vi "Sobel.vi"() -> ()   [LabVIEW 2015]
uses:
  <vilib>/vision/NI_Vision_Development_Module.lvlib
panel:
  in  "Threshold":sgl(slide) scale=0.0..10.0
  in  "index":u8(slide) scale=-1.0..8.0
  out "Sobel":T1(plugin-control)
  out "Source":T1(plugin-control)
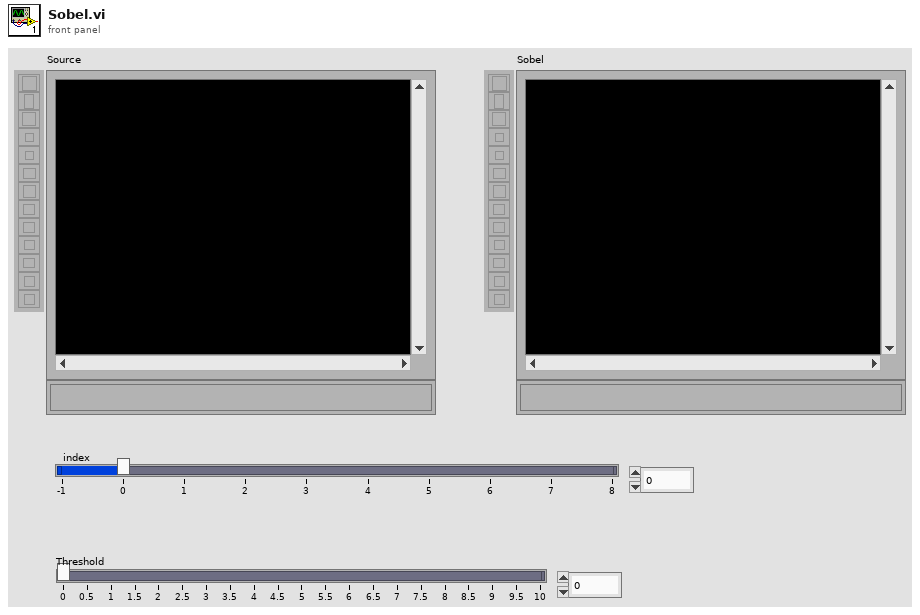
[diagram p1: front panel]
types:
  T1 = typedef "IMAQ Image.ctl" = refnum<image>
  T2 = enum32{"Differentiation", "Gradient", "Prewitt", "Roberts", "Sigma", "Sobel"}
  T3 = typedef "Image Type" = u32
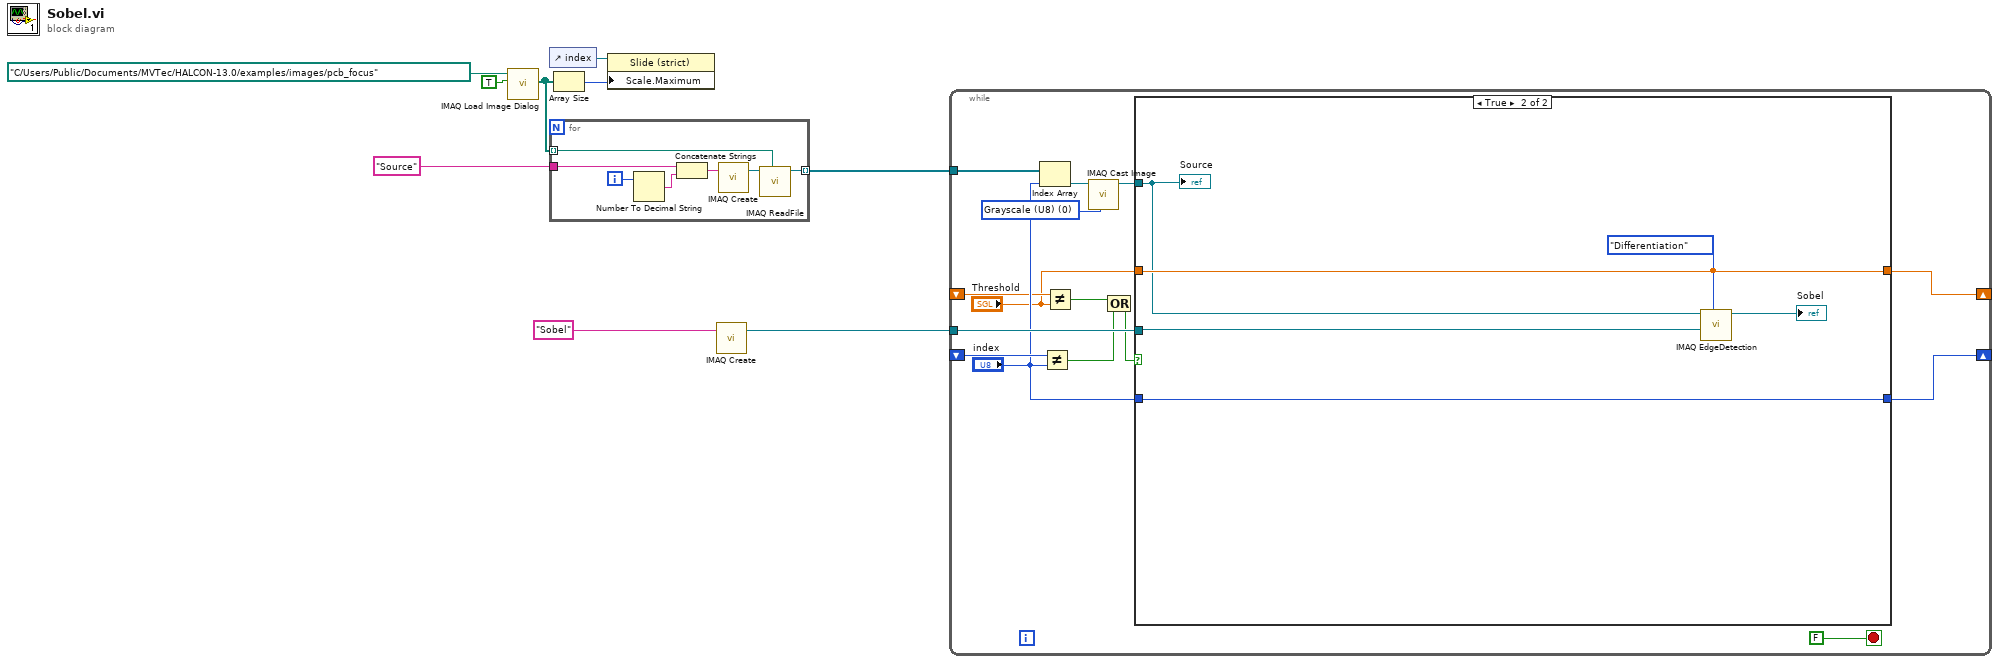
[diagram p0: block diagram]
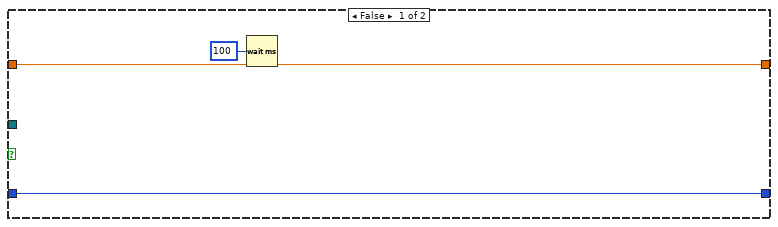
[diagram p2: hidden frame]
diagram:
  n1 = call "IMAQ Load Image Dialog"("Multiple Files? (No)"=TRUE, "Start Path"=path "C:/Users/Public/Documents/MVTec/HALCON-13.0/examples/images/pcb_focus") -> ("Paths"=w4:path[])  [unwired: 7 in, 2 out]
  n2 = control-ref of="index"() -> (w5:refnum<vi>)
  n3 = for {
    tunnel: w4 -> [w16] mode=indexing
    tunnel: "Source" ("Image Name") -> [w13]
    tunnel: [w10] -> w2 mode=indexing
    i -> [w14]
    n4 = Number To Decimal String(number=w14) -> (decimal integer string=w12:string)  [unwired: 1 in]
    n5 = Concatenate Strings(w13, w12) -> (w11:string)
    n6 = call "IMAQ Create"("Image Name"=w11) -> ("New Image"=w15:T1)  [unwired: 4 in, 1 out]
    n7 = call "IMAQ ReadFile"("File Path"=w16, "Image"=w15) -> ("Image Out"=w10:T1)  [unwired: 5 in, 4 out]
  }
  n8 = Array Size(array=w4) -> (size(s)=w3:i32)
  n9 = property class="Slide (strict)"(reference=w5, "Scale.Maximum"=w3) -> ()  [unwired: 1 in, 2 out]
  n10 = call "IMAQ Create"("Image Name"="Sobel") -> ("New Image"=w8:T1)  [unwired: 4 in, 1 out]
  n11 = while {
    tunnel: w8 -> [w31]
    tunnel: w2 -> [w29]
    shift-right: [w26] -> _
    shift-left: _ -> [w28]
    shift-right: [w25] -> _
    shift-left: _ -> [w24]
    stop <- FALSE stop-if-true
    w18 = T3 0 items=["Grayscale (U8)", "Grayscale (I16)", "Grayscale (SGL)", "Complex (CSG)", "RGB (U32)", "HSL (U32)", "RGB (U64)", "Grayscale (U16)"] ("Image Type")
    n12 = Index Array(array=w29, index="index") -> (element=w17:T1)
    n13 = Not Equal?(x=w28, y="index") -> (x != y?=w21:bool)
    n14 = Not Equal?(x=w24, y="Threshold") -> (x != y?=w22:bool)
    n15 = call "IMAQ Cast Image"("Image Type"=w18, "Image Src"=w17) -> ("Image Dst Out"=w19:T1)  [unwired: 8 in, 1 out]
    n16 = Compound Arithmetic op=OR(w22, w21) -> (w20:bool)
    n17 = case shown="True" w20 {
      tunnel: w19 -> [_ w35]
      tunnel: w31 -> [_ w36]
      tunnel: "index" -> [w34 w40]
      tunnel: [w34 w40] -> w26
      tunnel: [w32 w37] -> w25
      tunnel: "Threshold" -> [w32 w37]
      frame False {
        n18 = Wait (ms)(milliseconds to wait=u32 100) -> ()  [unwired: 1 out]
      }
      frame True {
        n19 = call "IMAQ EdgeDetection"("Method"=T2."Differentiation", "Threshold Value"=w37, "Image Dst"=w36, "Image Src"=w35) -> ("Image Dst Out"=→"Sobel":T1)  [unwired: 6 in, 1 out]
        "Source" <- w35
      }
    }
  }
